vi "Write Mode for Deleting Stale Data.vi"(8 "error in (no error)":errorcluster, 10 "delete stale samples when":T1, 11 "Waveforms (N Ch) in":refnum<class "Waveforms (N Ch).lvclass">) -> (0 "error out":errorcluster, 3 "Waveforms (N Ch) out":refnum<class "Waveforms (N Ch).lvclass">)   [LabVIEW 2017, in "Waveforms (N Ch).lvclass"]
uses:
  <vilib>/addons/_NISVFA/_Shared subVIs/Data Objects/Waveforms (DBL)/Waveforms (N Ch).lvclass
  C:/Program Files (x86)/National Instruments/LabVIEW 2017/vi.lib/addons/_NISVFA/_Shared subVIs/Data Objects/Data/Data.lvclass
  <vilib>/addons/_NISVFA/_Shared subVIs/Controls/svc_Delete Data Options (enum).ctl
  <vilib>/addons/_NISVFA/_Shared subVIs/Data Objects/Data/Data.lvclass/Data.ctl
  <vilib>/addons/_NISVFA/_Shared subVIs/Data Objects/Data/Data.lvclass
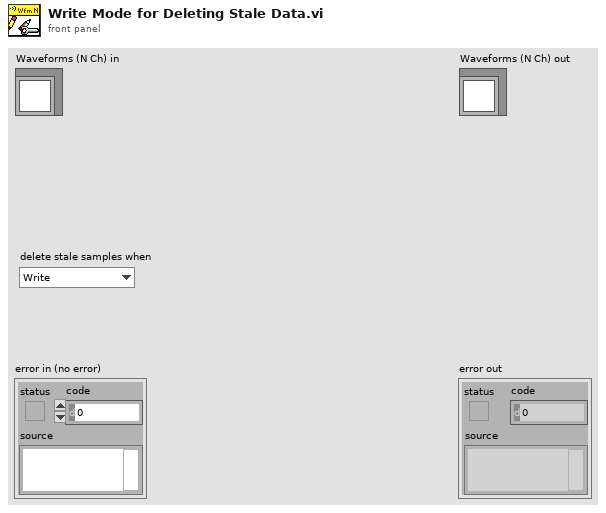
[diagram p1: front panel]
types:
  T1 = typedef "svc_Delete Data Options (enum).ctl" = enum16{"Write", "Read", "Release"}
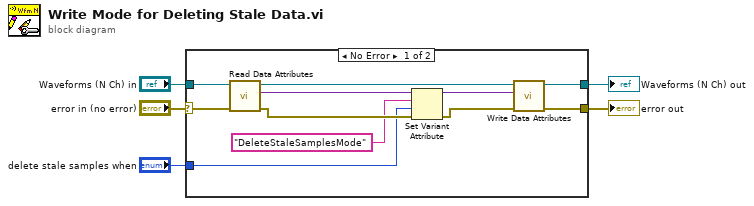
[diagram p0: block diagram]
diagram:
  n1 = case shown="No Error" "error in (no error)" {
    selector: "error in (no error)" -> [w12 w17]
    tunnel: [w9 w17] -> w4
    tunnel: [w15 w18] -> w2
    tunnel: "Waveforms (N Ch) in" -> [w6 w18]
    tunnel: "delete stale samples when" -> [w8 _]
    frame No Error {
      n2 = call <vilib>:"Read Data Attributes.vi"("error in (no error)"=w12, "Data in"=w6) -> ("error out"=w11:errorcluster, "data attributes"=w14:variant, "Data out"=w16:refnum<class "Waveforms (N Ch).lvclass">)  [unwired: 7 in]
      n3 = Set Variant Attribute(Variant=w14, name="DeleteStaleSamplesMode", value=w8, error in=w11) -> (Variant out=w13:variant, error out=w10:errorcluster)  [unwired: 1 out]
      n4 = call <vilib>:"Write Data Attributes.vi"("error in (no error)"=w10, "data attributes"=w13, "Data in"=w16) -> ("error out"=w9:errorcluster, "Data out"=w15:refnum<class "Waveforms (N Ch).lvclass">)  [unwired: 7 in]
    }
    frame Error {
    }
  }
  "error out" <- w4
  "Waveforms (N Ch) out" <- w2
